vi "CreateExecuteCommand.vi"   [LabVIEW 2017]
uses:
  <vilib>/Utility/miscctls.llb/LVPointTypeDef.ctl
types:
  T1 = typedef "LVPointTypeDef.ctl" = cluster{"Horizontal":i16, "Vertical":i16}
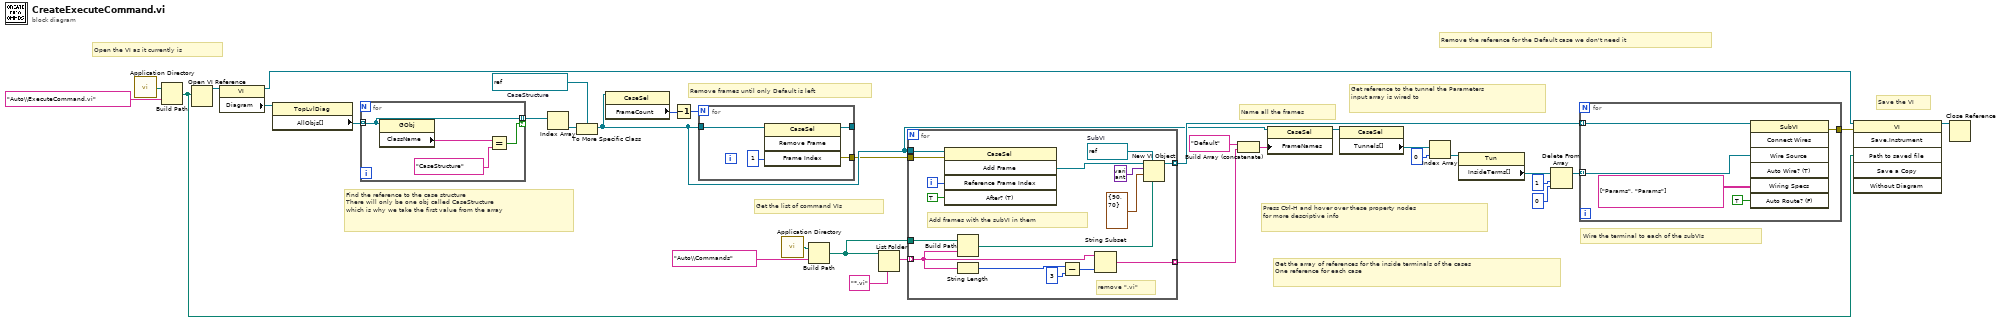
[diagram p0: block diagram]
diagram:
  w31 = refnum<vi> refnum  # CaseStructure
  # "Save the VI"
  # "Remove the reference for the Default case we don't need it"
  # "Get the array of references for the inside terminals of the cases\nOne reference for each case"
  # "Get reference to the tunnel the Parameters\ninput array is wired to"
  # "Press Ctrl-H and hover over these property nodes\nfor more descriptive info"
  # "Wire the terminal to each of the subVIs"
  # "Name all the frames"
  # "Get the list of command VIs"
  # "Remove frames until only Default is left"
  # "Find the reference to the case structure\nThere will only be one obj called CaseStructure\nwhich is why we take the first value from the array"
  # "Open the VI as it currently is"
  n1 = call <vilib>:"Application Directory.vi"() -> ("Application Directory"=w15:path)
  n2 = Build Path(base path=w15, name or relative path="Auto\\ExecuteCommand.vi") -> (appended path=w6:path)
  n3 = Open VI Reference(vi path=w6) -> (vi reference=w9:refnum<vi>)  [unwired: 5 in, 1 out]
  n4 = property class="VI"(reference=w9) -> (reference out=w8:refnum<vi>, "Diagram"=w10:refnum<vi>)  [unwired: 1 in, 1 out]
  n5 = property class="TopLvlDiag"(reference=w10) -> ("AllObjs[]"=w25:refnum<vi>[])  [unwired: 1 in, 2 out]
  n6 = for {
    tunnel: w25 -> [w34] mode=indexing
    tunnel: [w34] -> w33 mode=indexing if=w35
    n7 = property class="GObj"(reference=w34) -> ("ClassName"=w37:string)  [unwired: 1 in, 2 out]
    n8 = Equal?(x=w37, y="CaseStructure") -> (x = y?=w35:bool)
  }
  n9 = Index Array(array=w33) -> (element=w32:refnum<vi>)  [unwired: 1 in]
  n10 = To More Specific Class(target class=w31, reference=w32) -> (specific class reference=w2:refnum<vi>)  [unwired: 1 in, 1 out]
  n11 = property class="CaseSel"(reference=w2) -> ("FrameCount"=w4:i32)  [unwired: 1 in, 2 out]
  n12 = Decrement(x=w4) -> (x-1=w3:i32)
  n13 = for {
    N: w3 -> [_]
    tunnel: w2 -> [w41]
    tunnel: [w40] -> _
    tunnel: [w38] -> w1
    n14 = invoke class="CaseSel" method="Remove Frame"(reference=w41, "Frame Index"=u32 1) -> (reference out=w40:refnum<vi>, error out=w38:errorcluster)  [unwired: 2 in, 2 out]
  }
  n15 = call <vilib>:"Application Directory.vi"() -> ("Application Directory"=w12:path)
  n16 = Build Path(base path=w12, name or relative path="Auto\\Commands") -> (appended path=w11:path)
  n17 = List Folder(path=w11, pattern="*.vi") -> (filenames=w29:string[])  [unwired: 2 in, 3 out]
  n18 = for {
    tunnel: w2 -> [w56]
    tunnel: w29 -> [w47] mode=indexing
    tunnel: [w43] -> w28 mode=indexing
    tunnel: w11 -> [w55]
    tunnel: [w48] -> w21 mode=indexing
    tunnel: w1 -> [w42]
    i -> [w50]
    w53 = refnum<vi> refnum  # SubVI
    # "Add frames with the subVI in them"
    # "remove \".vi\""
    n19 = invoke class="CaseSel" method="Add Frame"(reference=w56, error in=w42, "Reference Frame Index"=w50, "After? (T)"=TRUE) -> ("Add Frame"=w49:refnum<vi>)  [unwired: 1 in, 4 out]
    n20 = Build Path(base path=w55, name or relative path=w47) -> (appended path=w54:path)
    n21 = String Length(string=w47) -> (length=w46:i32)
    n22 = Subtract(x=w46, y=3) -> (x-y=w44:i32)
    n23 = String Subset(string=w47, length (rest)=w44) -> (substring=w43:string)  [unwired: 1 in]
    n24 = New VI Object(vi object class=w53, owner refnum=w49, style=variant, position/next to=T1 {"Horizontal"=90, "Vertical"=70} ("location"), 6:w54) -> (object refnum=w48:refnum<vi>)  [unwired: 3 in, 1 out]
  }
  n25 = Build Array (concatenate)("Default", w28) -> (w27:string[])
  n26 = property class="CaseSel"(reference=w2, "FrameNames"=w27) -> (reference out=w20:refnum<vi>)  [unwired: 1 in, 1 out]
  n27 = property class="CaseSel"(reference=w20) -> ("Tunnels[]"=w22:refnum<vi>[])  [unwired: 1 in, 2 out]
  n28 = Index Array(array=w22, index=0) -> (element=w23:refnum<vi>)
  n29 = property class="Tun"(reference=w23) -> ("InsideTerms[]"=w19:refnum<vi>[])  [unwired: 1 in, 2 out]
  n30 = Delete From Array(array=w19, length=1, index=0) -> (array with subset deleted=w16:refnum<vi>[])  [unwired: 1 out]
  n31 = for {
    tunnel: w21 -> [w62] mode=indexing
    tunnel: w16 -> [w59] mode=indexing
    tunnel: [w58] -> w7
    n32 = invoke class="SubVI" method="Connect Wires"(reference=w62, "Wire Source"=w59, "Wiring Specs"=string[][] [["Params", "Params"]], "Auto Route? (F)"=TRUE) -> (error out=w58:errorcluster)  [unwired: 3 in, 6 out]
  }
  n33 = invoke class="VI" method="Save.Instrument"(reference=w8, error in=w7, "Path to saved file"=w6) -> (reference out=w5:refnum<vi>)  [unwired: 3 in, 5 out]
  n34 = Close Reference(reference=w5) -> ()  [unwired: 1 in, 1 out]
